vi "Write Measurement Edge.vi"(8 "error in":errorcluster, 10 "measurement edge":T1, 11 "period measurement channel in":refnum<class "Period Measurement Channel.lvclass">) -> (0 "error out":errorcluster, 3 "period measurement channel out":refnum<class "Period Measurement Channel.lvclass">)   [LabVIEW 2017, in "Period Measurement Channel.lvclass"]
uses:
  Period Measurement Channel.lvclass
  Measurement Edge.ctl
  Period Measurement Channel.lvclass/Period Measurement Channel.ctl
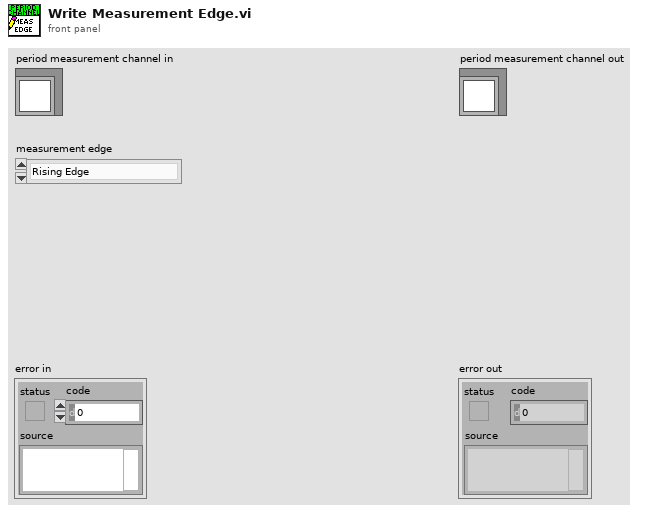
[diagram p1: front panel]
types:
  T1 = typedef "Period Measurement Channel.lvclass/Measurement Edge.ctl" = enum16{"Rising Edge", "Falling Edge"}
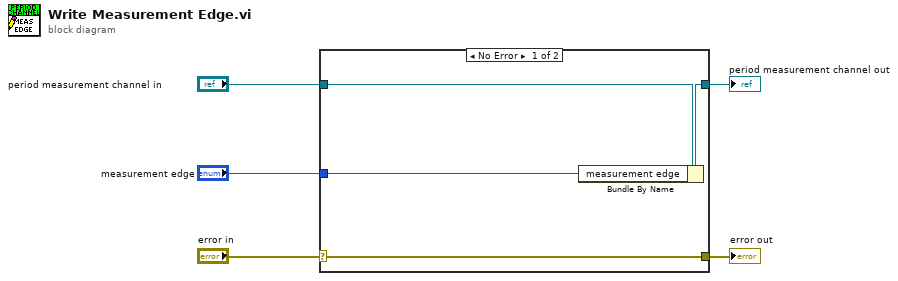
[diagram p0: block diagram]
diagram:
  n1 = case shown="No Error" "error in" {
    selector: "error in" -> [w9 w10]
    tunnel: [w9 w10] -> w4
    tunnel: [w7 w11] -> w2
    tunnel: "period measurement channel in" -> [w8 w11]
    tunnel: "measurement edge" -> [w6 _]
    frame No Error {
      n2 = Bundle By Name(cluster=w8, "measurement edge"=w6) -> (w7:refnum<class "Period Measurement Channel.lvclass">)
    }
    frame Error {
    }
  }
  "error out" <- w4
  "period measurement channel out" <- w2
